vi "Generate Trajectory.vi"(6 "Angular Accelerations":T1 {"Angular \nAccelerations" step=5.0}, 8 "Conditions":T3, 9 "Limits":T2={"Velocity (fps)"=6.0, "Acceleration (fps^2)"=15.0, "Jerk (fps^3)"=100.0}, 10 "WayPoints":cluster{"x":dbl, "y":dbl, "th":dbl}[](array[cluster]), 11 "Sample Period (s)":dbl=0.02) -> (0 "Updated Waypoints":cluster{"x":dbl, "y":dbl, "th":dbl}[](array[cluster]), 1 "Valid":bool, 2 "Time (s)":dbl, 3 "Trajectory Data":T4(array[cluster]), 4 "Distance (ft)":dbl)   [LabVIEW 2018]
panel:
  # "TURN Acceleration"
  # "1"
  # "1"
  # "2"
  # "2"
  # "3"
  # "3"
  # "4"
  # "4"
  # "5"
  # "5"
  # "6"
  # "6"
  # "7"
  # "7"
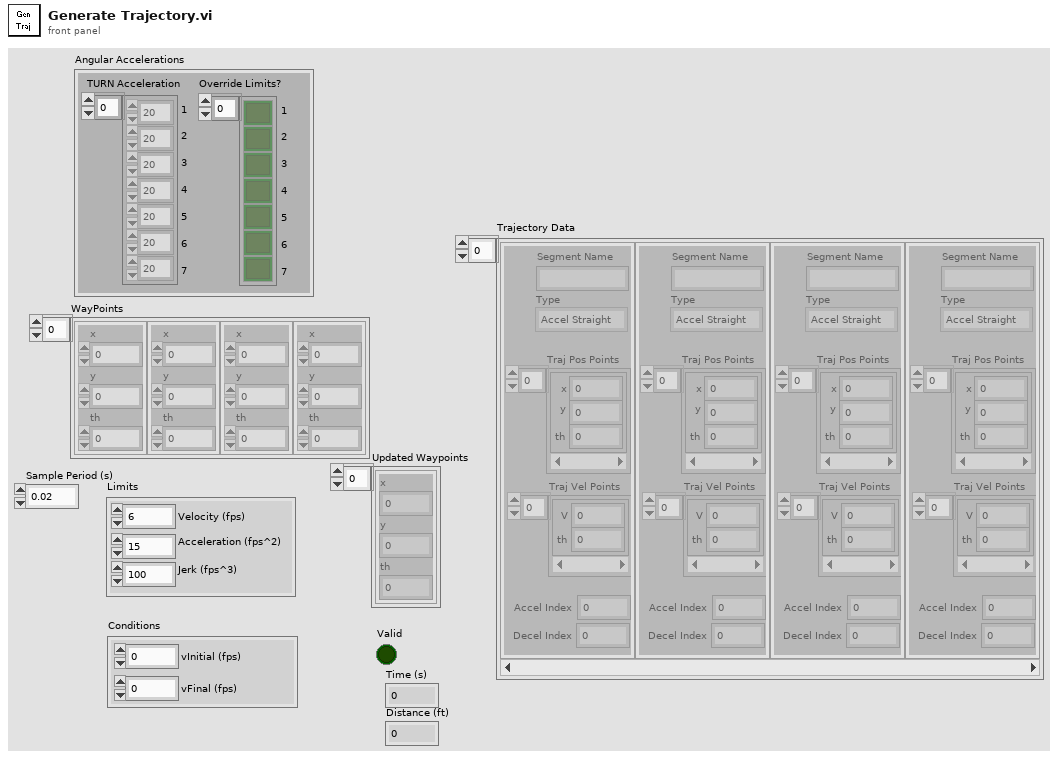
[diagram p1: front panel]
types:
  T1 = cluster{"Angular \nAccelerations":dbl[], "Override Limits?":bool[]}
  T2 = cluster{"Velocity (fps)":dbl, "Acceleration (fps^2)":dbl, "Jerk (fps^3)":dbl}
  T3 = cluster{"vInitial (fps)":dbl, "vFinal (fps)":dbl}
  T4 = cluster{"Segment Name":string, "Type":enum16{"Accel Straight", "Const Straight", "Blend", "Circle"}, "Traj Pos Points":cluster{"x":dbl, "y":dbl, "th":dbl}[], "Traj Vel Points":cluster{"V":dbl, "th":dbl}[], "Accel Index":i32, "Decel Index":i32}[]
  T5 = cluster{"distance (ft)":dbl, "dist of baseline Jerk":dbl, "dist of high Jerk":dbl}
  T6 = cluster{"Velocity (fps)":dbl, "Acceleration (fps^2)":dbl, "vInitial (fps)":dbl, "Sample Period (s)":dbl, "Jerk (fps^3)":dbl, cluster{"distance (ft)":dbl, "dist of baseline Jerk":dbl, "dist of high Jerk":dbl}, cluster{"distance (ft)":dbl, "dist of baseline Jerk":dbl, "dist of high Jerk":dbl}}
  T7 = cluster{"Point Out":cluster{"x":dbl, "y":dbl, "th":dbl}, "Point Out":cluster{"x":dbl, "y":dbl, "th":dbl}, "Valid":bool}[]
  T8 = typedef "BlendType.ctl" = cluster{"Scaling":dbl, "Length":dbl, "Angle":dbl, "Vertex Dist":dbl, "ParaTime":dbl, "ExtraArc":dbl, "Center Point":cluster{dbl, dbl}}
  T9 = cluster{"Velocity (fps)":dbl, "Velocity (fps)":dbl}
  T10 = cluster{"Segment Name":string, "Type":enum16{"Accel Straight", "Const Straight", "Blend", "Circle"}, "Traj Pos Points":cluster{"x":dbl, "y":dbl, "th":dbl}[], "Traj Vel Points":cluster{"V":dbl, "th":dbl}[], "Accel Index":i32, "Decel Index":i32}
  T11 = cluster{"maxV (fps)":dbl, "Accel Limit (fps^2)":dbl, "Initial V (fps)":dbl, "Sample Period (s)":dbl, "Jerk Limit (fps^3)":dbl, "Front Distances":cluster{"distance (ft)":dbl, "baseline (ft)":dbl, "high (ft)":dbl}, "Back Distances":cluster{"distance (ft)":dbl, "baseline (ft)":dbl, "high (ft)":dbl}}
  T12 = cluster{"maxV (fps)":dbl, "Accel Limit (fps^2)":dbl, "Initial V (fps)":dbl, "Sample Period (s)":dbl, "Jerk Limit (fps^3)":dbl, "Jerk Distances":cluster{"distance (ft)":dbl, dbl, dbl}, "Jerk Distances":cluster{"distance (ft)":dbl, dbl, dbl}}
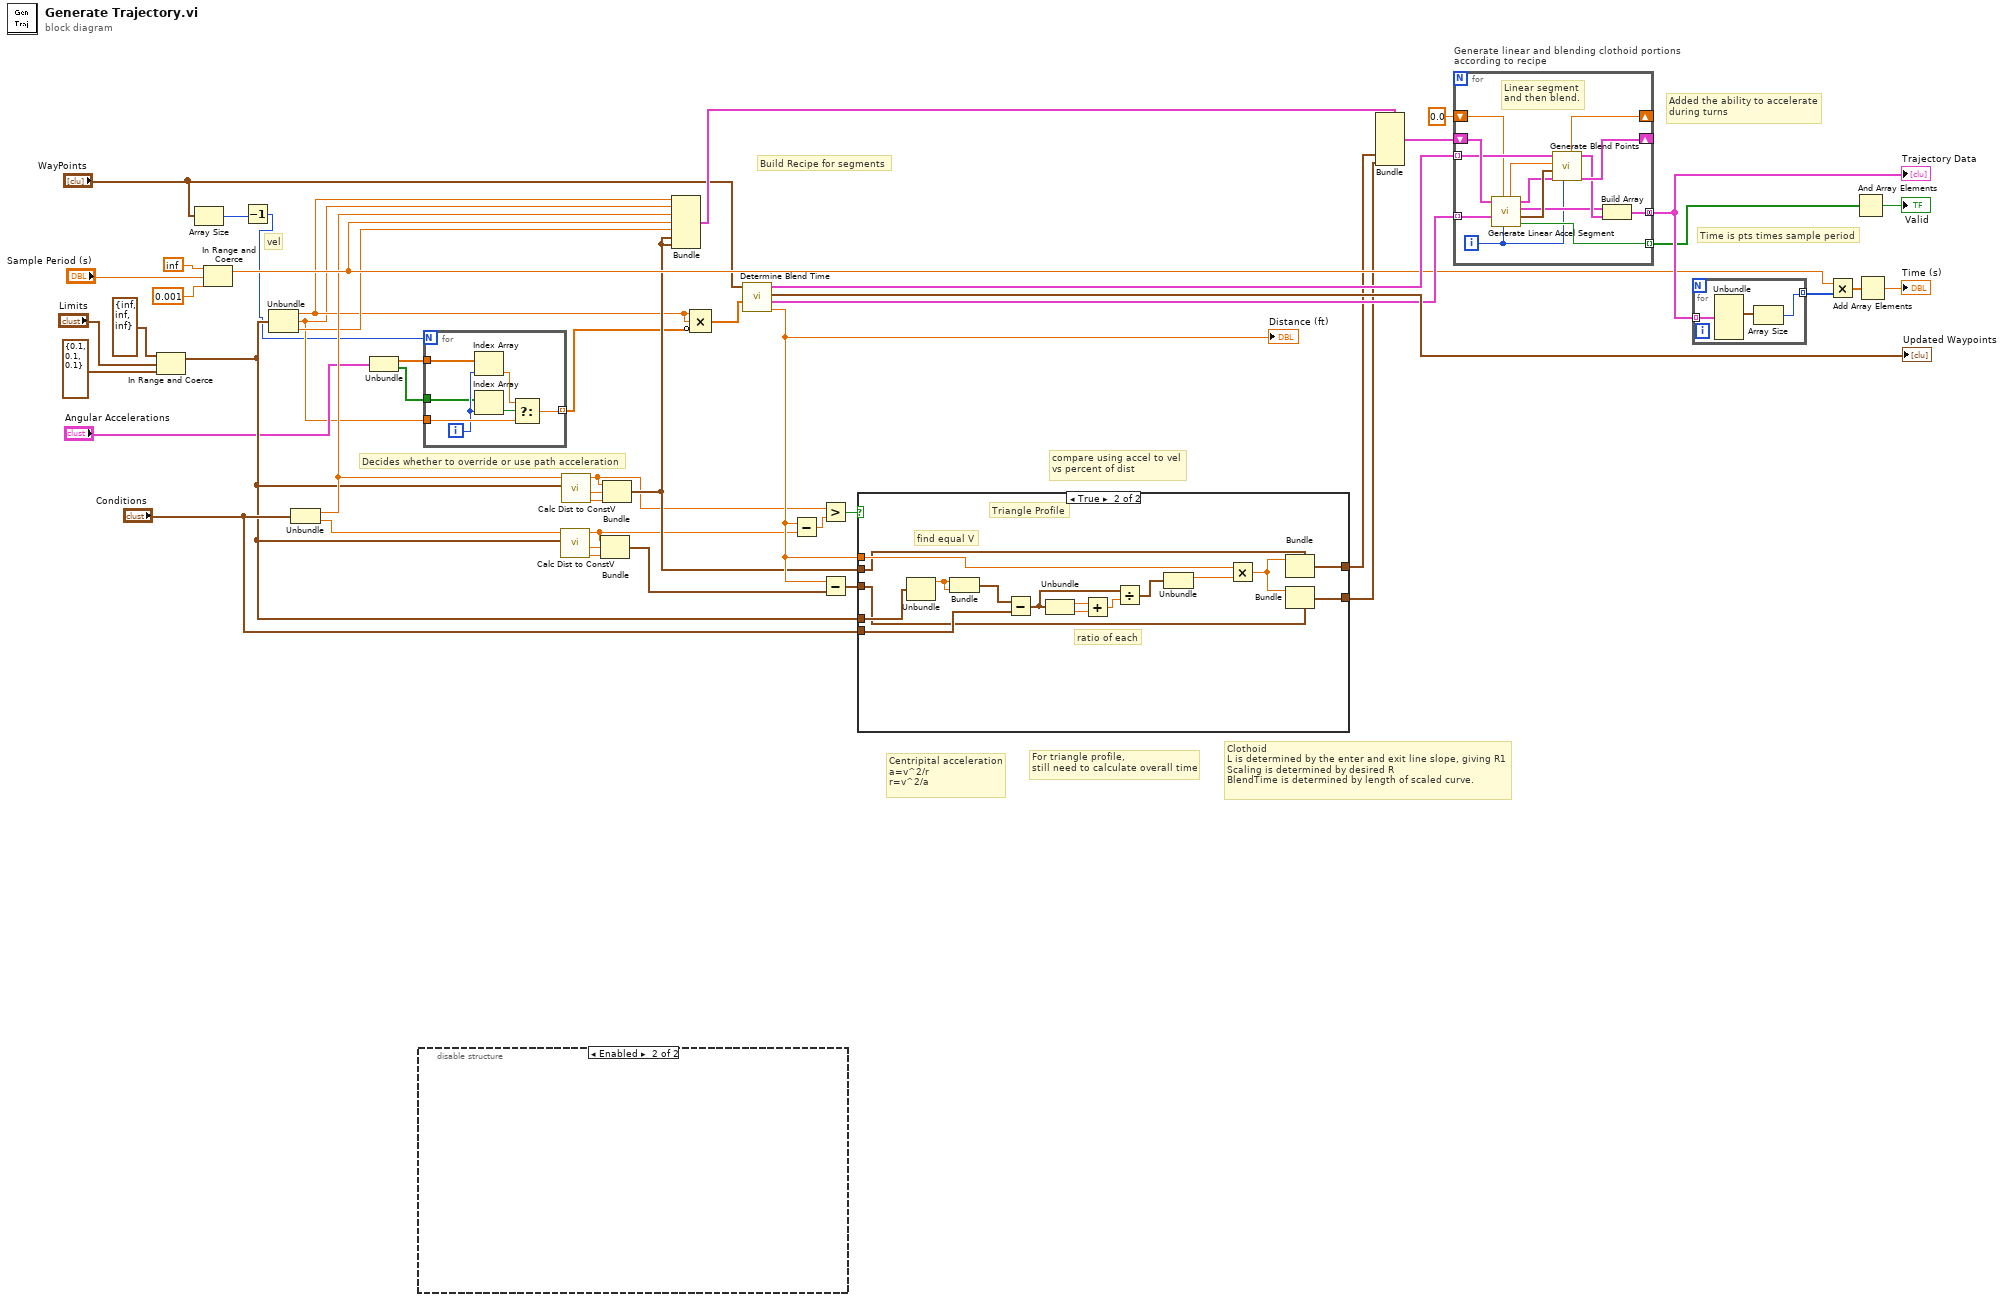
[diagram p0: block diagram]
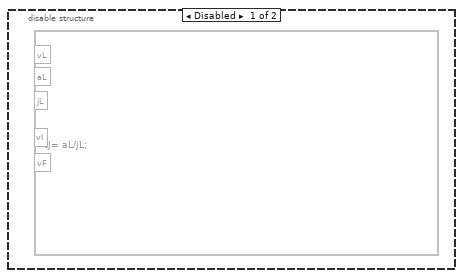
[diagram p2: hidden frame]
diagram:
  # "Added the ability to accelerate\nduring turns"
  # "Decides whether to override or use path acceleration"
  # "For triangle profile,\nstill need to calculate overall time"
  # "compare using accel to vel\nvs percent of dist"
  # "Build Recipe for segments"
  # "Time is pts times sample period"
  # "Clothoid\nL is determined by the enter and exit line slope, giving R1\nScaling is determined by desired R\nBlendTime is determined by length of scaled curve."
  # "Centripital acceleration\na=v^2/r\nr=v^2/a"
  # "vel"
  n1 = In Range and Coerce(upper limit=T2 {"Velocity (fps)"=inf, "Acceleration (fps^2)"=inf, "Jerk (fps^3)"=inf}, x="Limits", lower limit=T2 {"Velocity (fps)"=0.1, "Acceleration (fps^2)"=0.1, "Jerk (fps^3)"=0.1} ("upper limit")) -> (coerced(x)=w24:T2)  [unwired: 1 out]
  n2 = Array Size(array="WayPoints") -> (size(s)=w4:i32)
  n3 = In Range and Coerce(upper limit=inf, x="Sample Period (s)", lower limit=0.001) -> (coerced(x)=w34:dbl)  [unwired: 1 out]
  n4 = Decrement(x=w4) -> (x-1=w2:i32)
  n5 = Unbundle(w24) -> ("Velocity (fps)"=w11:dbl, "Acceleration (fps^2)"=w6:dbl, "Jerk (fps^3)"=w25:dbl)
  n6 = Unbundle("Conditions") -> ("vInitial (fps)"=w30:dbl, "vFinal (fps)"=w29:dbl)
  n7 = Unbundle("Angular Accelerations") -> ("Angular \nAccelerations"=w8:dbl[], "Override Limits?"=w7:bool[])
  n8 = disable-structure shown="Enabled" {
    frame Disabled {
      n9 = formula code="tJ= aL/jL;"() -> ()  [unwired: 5 in]
    }
    frame Enabled {
    }
  }
  n10 = for {
    N: w2 -> [_]
    tunnel: w8 -> [w53]
    tunnel: w7 -> [w50]
    tunnel: w6 -> [w55]
    tunnel: [w54] -> w5 mode=indexing
    i -> [w51]
    n11 = Index Array(array=w53, index=w51) -> (element=w52:dbl)
    n12 = Index Array(array=w50, index=w51) -> (element=w49:bool)
    n13 = Select(t=w52, s=w49, f=w55) -> (s? t:f=w54:dbl)
  }
  n14 = call "Calc Dist to ConstV.vi"("Limits"=w24, "V endpoint (fps)"=w29) -> ("dist of high Jerk"=w21:dbl, "dist of baseline Jerk"=w20:dbl, "distance (ft)"=w14:dbl)  [unwired: 6 in, 1 out]
  n15 = call "Calc Dist to ConstV.vi"("Limits"=w24, "V endpoint (fps)"=w30) -> ("dist of high Jerk"=w23:dbl, "dist of baseline Jerk"=w22:dbl, "distance (ft)"=w15:dbl)  [unwired: 6 in, 1 out]
  n16 = Bundle("distance (ft)"=w14, "dist of baseline Jerk"=w20, "dist of high Jerk"=w21) -> (w18:T5)  [unwired: 1 in]
  n17 = Bundle("distance (ft)"=w15, "dist of baseline Jerk"=w22, "dist of high Jerk"=w23) -> (w16:T5)  [unwired: 1 in]
  n18 = Bundle("Velocity (fps)"=w11, "Acceleration (fps^2)"=w6, "vInitial (fps)"=w30, "Sample Period (s)"=w34, "Jerk (fps^3)"=w25, w16, w16) -> (w36:T6)  [unwired: 1 in]
  n19 = Compound Arithmetic op=MULTIPLY(w11, w11, invert w5) -> (w10:dbl[])
  n20 = call "Determine Blend Time.vi"("Min R"=w10, "WayPoints"="WayPoints") -> ("Distance"=w19:dbl, "Linear Info"=w45:T7, "Updated Waypoints"=→"Updated Waypoints":cluster{"x":dbl, "y":dbl, "th":dbl}[], "Blends"=w44:T8[])  [unwired: 6 in]
  "Distance (ft)" <- w19
  n21 = Subtract(x=w19, y=w14) -> (x-y=w26:dbl)
  n22 = Greater?(x=w15, y=w26) -> (0:w28:bool)
  n23 = Subtract(x=w19, y=w18) -> (x-y=w17:T5)
  n24 = case shown="True" w28 {
    tunnel: w24 -> [_ w73]
    tunnel: "Conditions" -> [_ w70]
    tunnel: w19 -> [_ w60]
    tunnel: w16 -> [w57 w59]
    tunnel: [w57 w63] -> w13
    tunnel: w17 -> [w56 w58]
    tunnel: [w56 w62] -> w12
    frame False {
      # "Trapezoid Profile"
    }
    frame True {
      # "Triangle Profile"
      # "ratio of each"
      # "find equal V"
      n25 = Unbundle(w73) -> ("Velocity (fps)"=w72:dbl)  [unwired: 2 out]
      n26 = Bundle("Velocity (fps)"=w72, "Velocity (fps)"=w72) -> (w71:T9)  [unwired: 1 in]
      n27 = Subtract(x=w71, y=w70) -> (x-y=w67:cluster{dbl, dbl})
      n28 = Unbundle(w67) -> (w69:dbl, w68:dbl)
      n29 = Add(x=w69, y=w68) -> (x+y=w66:dbl)
      n30 = Divide(x=w67, y=w66) -> (x/y=w65:cluster{dbl, dbl})
      n31 = Unbundle(w65) -> (w64:dbl)  [unwired: 1 out]
      n32 = Multiply(x=w60, y=w64) -> (x*y=w61:dbl)
      n33 = Bundle(cluster=w59, "distance (ft)"=w61) -> (w63:T5)  [unwired: 2 in]
      n34 = Bundle(cluster=w58, "distance (ft)"=w61) -> (w62:T5)  [unwired: 2 in]
    }
  }
  n35 = Bundle(cluster=w36, w13, w12) -> (w35:T6)  [unwired: 5 in]
  n36 = for "Generate linear and blending clothoid portions\naccording to recipe" {
    tunnel: [w87] -> w41 mode=concatenating
    tunnel: w44 -> [w79] mode=indexing
    shift-right: [w86] -> _
    shift-left: w35 -> [w85]
    tunnel: w45 -> [w80] mode=indexing
    tunnel: [w78] -> w39 mode=indexing
    shift-right: [w75] -> _
    shift-left: 0.0 ("Final Acceleration") -> [w74]
    i -> [w77]
    # "Linear segment\nand then blend."
    n37 = call "Generate Linear Accel Segment.vi"("Index"=w77, "Initial Acceleration"=w74, "Linear Info"=w80, "Speeds"=w85) -> ("Valid"=w78:bool, "Final Position"=w84:cluster{dbl, dbl, dbl}, "Trajectory Segment"=w82:T10, "Speeds Out"=w81:T11, "Final Acceleration"=w76:dbl)  [unwired: 3 in]
    n38 = call "Generate Blend Points.vi"("Index"=w77, "Speeds"=w81, "Initial Point"=w84, "Initial Acceleration"=w76, "Blend Info"=w79) -> ("Speeds Out"=w86:T12, "Trajectory Segment"=w83:T10, "Final Acceleration"=w75:dbl)  [unwired: 4 in]
    n39 = Build Array(w82, w83) -> (w87:T4)
  }
  "Trajectory Data" <- w41
  n40 = for {
    tunnel: w41 -> [w90] mode=indexing
    tunnel: [w89] -> w43 mode=indexing
    n41 = Unbundle(w90) -> ("Traj Pos Points"=w88:cluster{"x":dbl, "y":dbl, "th":dbl}[])  [unwired: 5 out]
    n42 = Array Size(array=w88) -> (size(s)=w89:i32)
  }
  n43 = Multiply(x=w34, y=w43) -> (x*y=w42:dbl[])
  n44 = And Array Elements(Boolean array=w39) -> (logical AND=→"Valid":bool)
  n45 = Add Array Elements(numeric array=w42) -> (sum=→"Time (s)":dbl)
